vi "GV NpixelclockPerLine.vi"() -> ()   [LabVIEW 2017]
panel:
  out "NpixelclockPerLine":i16
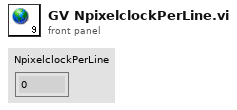
[diagram p1: front panel]
diagram:
